vi "Main.vi"() -> ()   [LabVIEW 2017]
doc: "The myRIO Project template acquires acceleration data from the onboard accelerometer and displays the changes of acceleration values in a waveform chart."
uses:
  <vilib>/myRIO/Instrument Drivers/Onboard IO/DIO/typedefs/DIO Reference.ctl
  <vilib>/myRIO/Common/Instrument Driver Framework/Utilities/typedefs/myRIO Generic Hardware Reference.ctl
  <vilib>/myRIO/Common/Instrument Driver Framework/Utilities/typedefs/Hardware Version Enum.ctl
  <vilib>/myRIO/Common/Instrument Driver Framework/Utilities/typedefs/myRIO v1.0 Reference.ctl
  <vilib>/myRIO/Common/Instrument Driver Framework/Utilities/typedefs/Generic FPGA Reference.ctl
  <vilib>/myRIO/Common/Instrument Driver Framework/myRIO v1.0/DIO/typedefs/DIO Channels List.ctl
  <vilib>/myRIO/Common/Instrument Driver Framework/myRIO v1.0/DIO/typedefs/DIO Channels Enum.ctl
  <vilib>/userdefined/High Color/nirio_resource_hc.ctl
  <vilib>/myRIO/Common/Instrument Driver Framework/Utilities/vis/Is FPGA Ref Available.vi
  <vilib>/myRIO/Common/Instrument Driver Framework/myRIO v1.0/DIO/vis/myRIO v1.1 Open DIO.vi
  <vilib>/myRIO/Instrument Drivers/Onboard IO/DIO/vis/Read.vi
  <vilib>/myRIO/Instrument Drivers/Onboard IO/DIO/vis/Write.vi
  <vilib>/myRIO/Common/Instrument Driver Framework/Utilities/vis/Validate Channels.vi
  <vilib>/myRIO/Common/Instrument Driver Framework/myRIO v1.0/DIO/vis/myRIO v1.0 Reserve DIO.vi
  <vilib>/myRIO/Common/Instrument Driver Framework/myRIO v1.0/Resource Manager/vis/myRIO v1.0 Reserve Channel List.vi
  <vilib>/myRIO/Common/Instrument Driver Framework/myRIO v1.0/DIO/vis/myRIO v1.0 Build MUX Configuration DIO.vi
  <vilib>/myRIO/Common/Instrument Driver Framework/myRIO v1.0/Resource Manager/vis/myRIO v1.0 Reserve Channel.vi
  <vilib>/myRIO/Common/Instrument Driver Framework/myRIO v1.0/Resource Manager/vis/myRIO v1.0 Unreserve Channel.vi
  <vilib>/myRIO/Common/Instrument Driver Framework/myRIO v1.0/Resource Manager/vis/myRIO v1.0 Create Configuration List.vi
  <vilib>/myRIO/Common/Instrument Driver Framework/myRIO v1.0/Resource Manager/vis/myRIO v1.0 Build Mutex Name.vi
  Constant.vi
  <vilib>/Utility/VariantDataType/GetNumericInfo.vi
  <vilib>/Utility/error.llb/Error Cluster From Error Code.vi
  <vilib>/myRIO/Common/Instrument Driver Framework/myRIO v1.0/myRIO v1.1 Open.vi
  <vilib>/myRIO/Common/Instrument Driver Framework/Utilities/vis/IO Manager.vi
  <vilib>/myRIO/Common/Instrument Driver Framework/Utilities/vis/Configuration Manager.vi
  <vilib>/myRIO/Common/Instrument Driver Framework/myRIO v1.0/Resource Manager/vis/myRIO v1.0 Configure IO.vi
  <vilib>/myRIO/Common/Instrument Driver Framework/myRIO v1.0/myRIO v1.0 Close.vi
  <vilib>/myRIO/Common/Instrument Driver Framework/myRIO v1.0/DIO/vis/myRIO v1.0 Write DIO.vi
  <vilib>/myRIO/Common/Instrument Driver Framework/myRIO v1.0/DIO/vis/myRIO v1.0 Read DIO.vi
  <vilib>/myRIO/Express VI/Onboard Devices/LED/LED Express VI.xnode
  <vilib>/myRIO/Instrument Drivers/Onboard IO/DIO/vis/myRIO DIO Open.xnode
  <vilib>/myRIO/Express VI/Onboard Devices/Button/Button Express VI.xnode
  <vilib>/myRIO/Instrument Drivers/Onboard IO/DIO/DIO.lvlib
panel:
  out "power":i8
  out "b_pos":i32
  out "f_pos":i32
  out "R_pos":i32
  out "L_pos":i32
  in  "Stop Button":bool
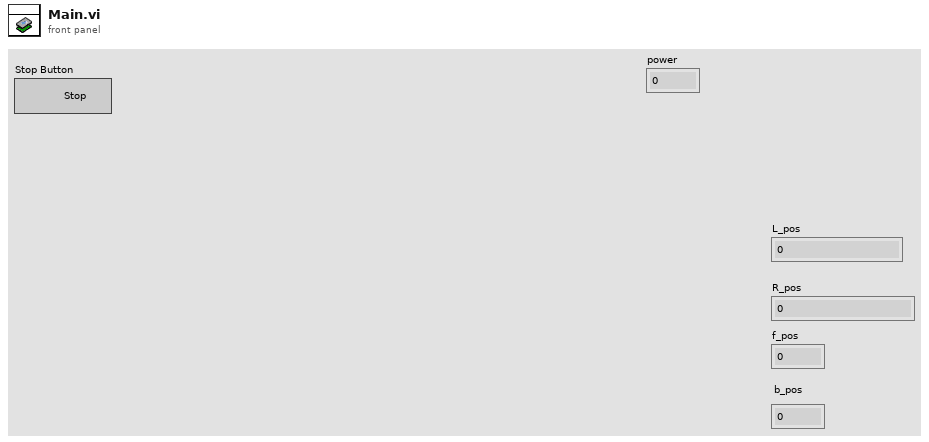
[diagram p1: front panel]
types:
  T1 = typedef "DIO.lvlib/DIO Reference.ctl" = cluster{"myRIO Reference":T2, "DIO Channels List":T6}
  T2 = typedef "myRIO Generic Hardware Reference.ctl" = cluster{"myRIO Model":T3, "myRIO Hardware Reference":T4}
  T3 = typedef "Hardware Version Enum.ctl" = enum16{"Unknown", "myRIO-1900", "myRIO-1950", "roboRIO", "NI ELVIS RIO CM"}
  T4 = typedef "myRIO v1.0 Reference.ctl" = cluster{"Generic FPGA Reference":T5, "Allow multiple opens":bool}
  T5 = typedef "Generic FPGA Reference.ctl" = refnum<k20>
  T6 = typedef "DIO Channels List.ctl" = T7[]
  T7 = typedef "DIO Channels Enum.ctl" = enum16{"Not Connected", "C/DIO0", "C/DIO1", "C/DIO2", "C/DIO3", "C/DIO4", "C/DIO5", "C/DIO6", "C/DIO7", "A/DIO0", "A/DIO1", "A/DIO2", "A/DIO3", "A/DIO4", "A/DIO5", "A/DIO6", "A/DIO7", "A/DIO8", "A/DIO9", "A/DIO10", "A/DIO11", "A/DIO12", "A/DIO13", "A/DIO14", "A/DIO15", "B/DIO0", "B/DIO1", "B/DIO2", "B/DIO3", "B/DIO4", "B/DIO5", "B/DIO6", "B/DIO7", "B/DIO8", "B/DIO9", "B/DIO10", "B/DIO11", "B/DIO12", "B/DIO13", "B/DIO14", "B/DIO15", "LED0", "LED1", "LED2", "LED3", "Button0", "DIO/DIO0", "DIO/DIO1", "DIO/DIO2", "DIO/DIO3", "DIO/DIO4", "DIO/DIO5", "DIO/DIO6", "DIO/DIO7", "DIO/DIO8", "DIO/DIO9", "SPI/CS0", "SPI/CS1", "SPI/CS2", "SPI/CS3", "LED RADIO (Green)", "LED RADIO (Red)", "LED COMM (Green)", "LED COMM (Red)", "LED MODE (Green)", "LED MODE (Red)"}
  T8 = typedef "nirio_resource_hc.ctl" = tag
  T9 = enum16{"hold", "f", "fl", "fr", "l", "r", "b", "bl", "br"}
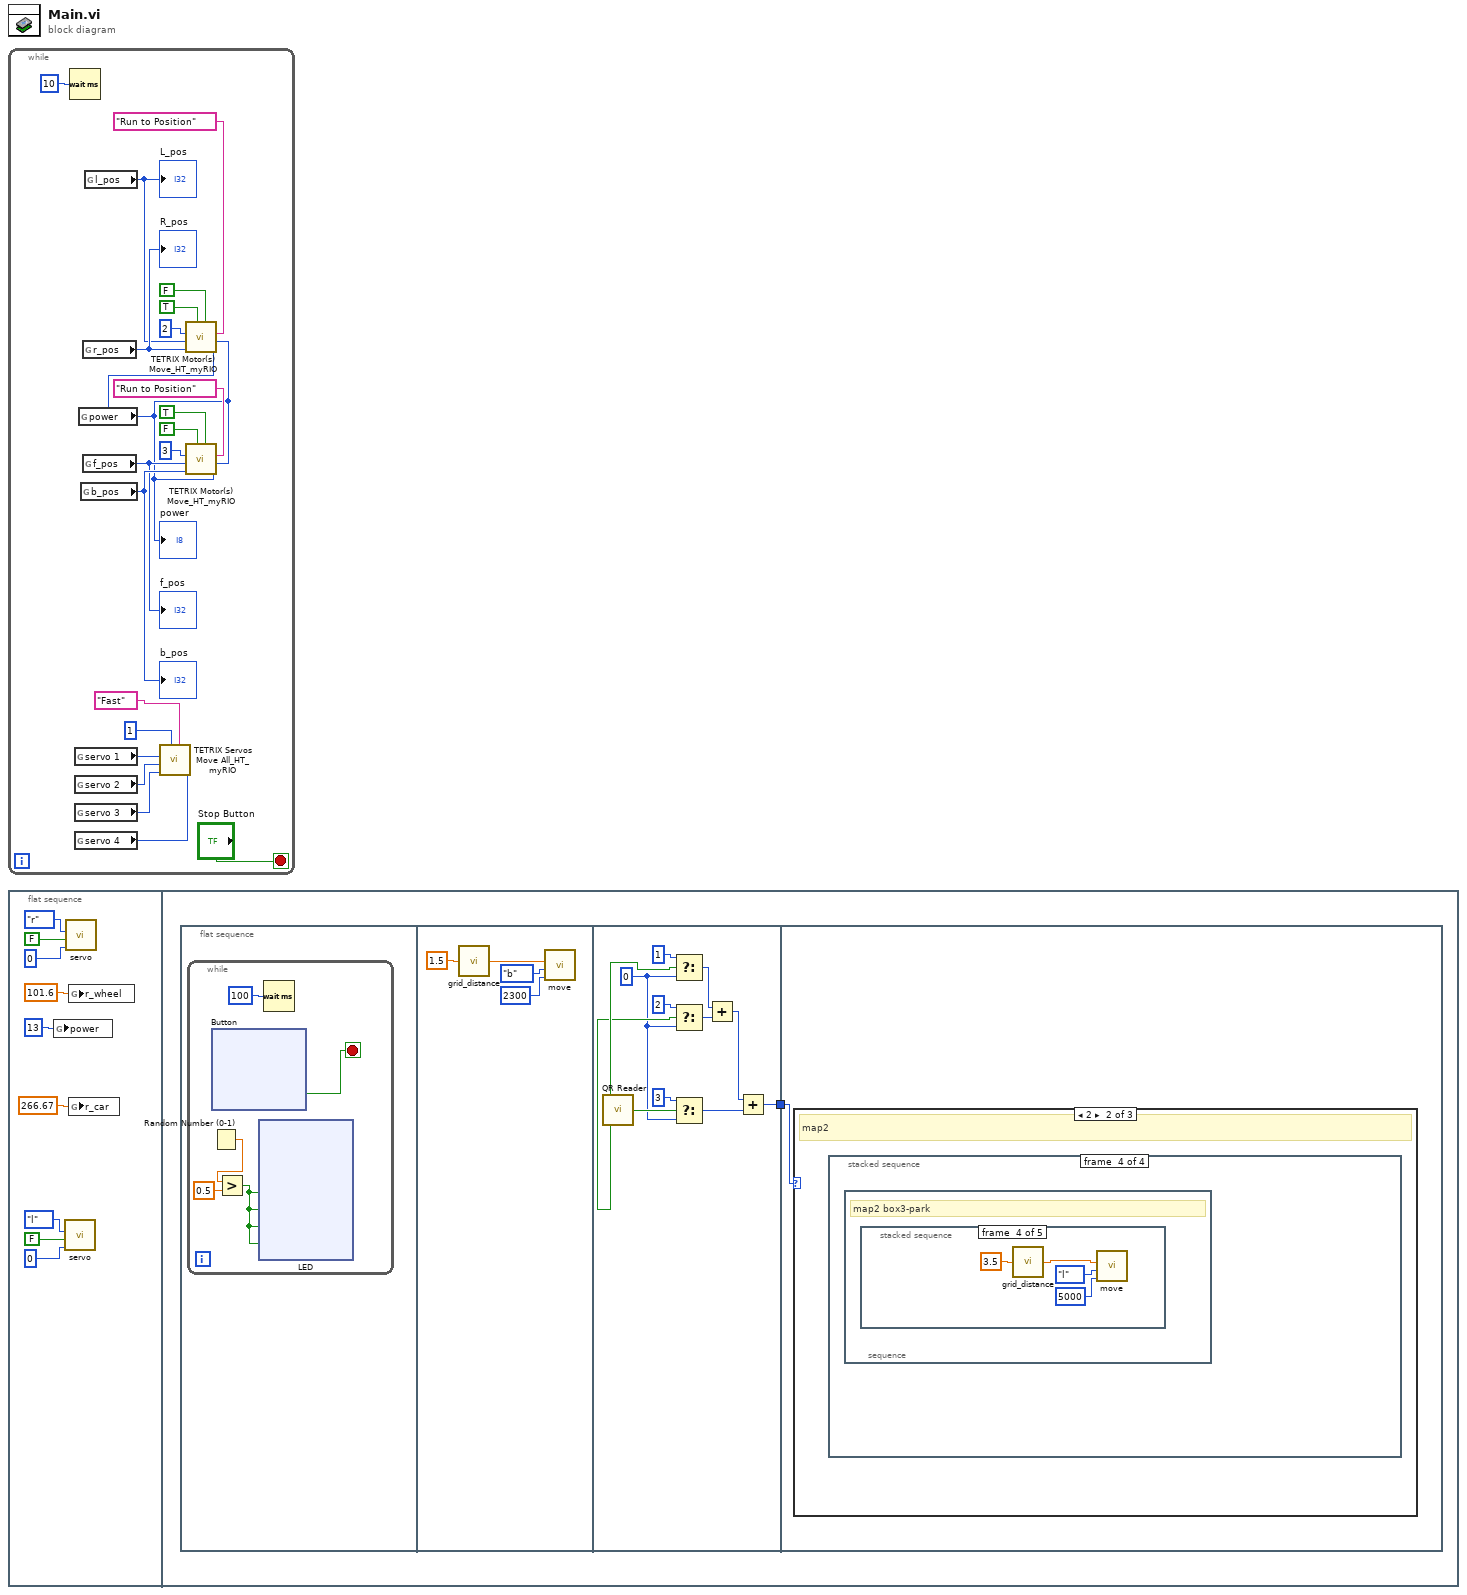
[diagram p0: block diagram]
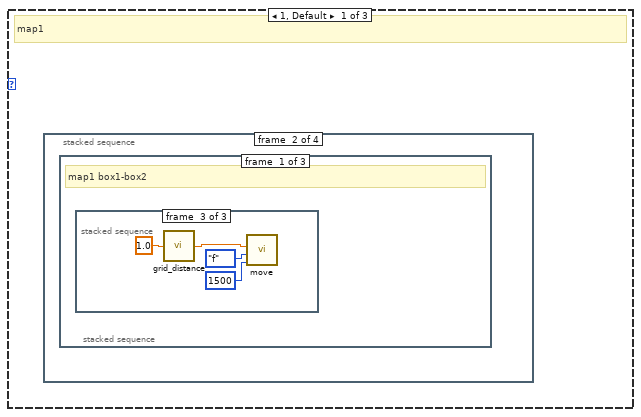
[diagram p2: hidden frame]
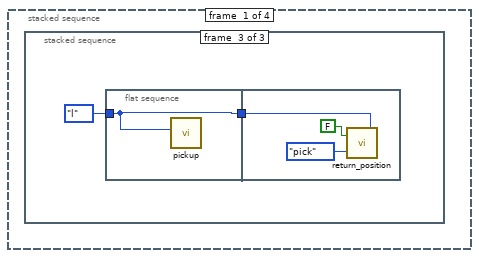
[diagram p3: hidden frame]
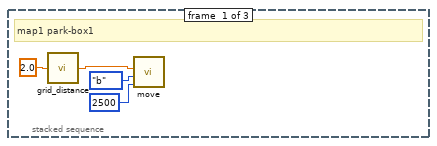
[diagram p4: hidden frame]
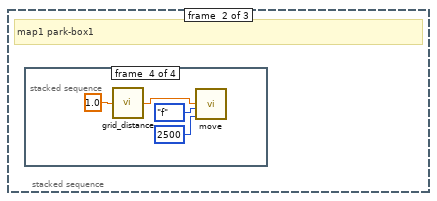
[diagram p5: hidden frame]
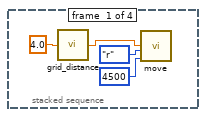
[diagram p6: hidden frame]
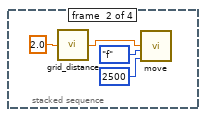
[diagram p7: hidden frame]
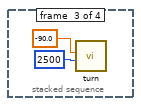
[diagram p8: hidden frame]
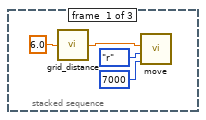
[diagram p9: hidden frame]
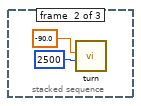
[diagram p10: hidden frame]
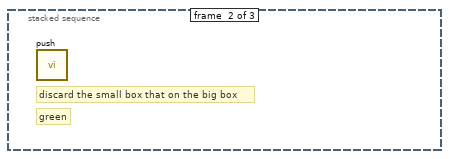
[diagram p11: hidden frame]
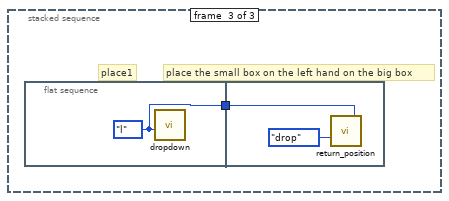
[diagram p12: hidden frame]
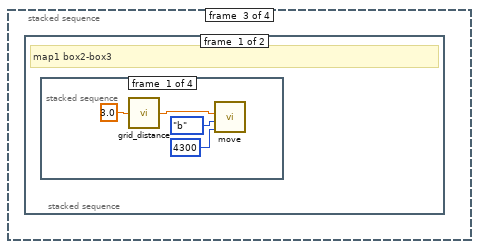
[diagram p13: hidden frame]
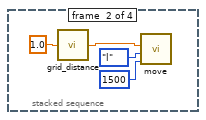
[diagram p14: hidden frame]
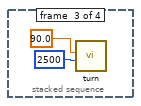
[diagram p15: hidden frame]
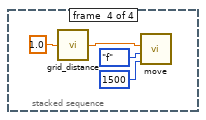
[diagram p16: hidden frame]
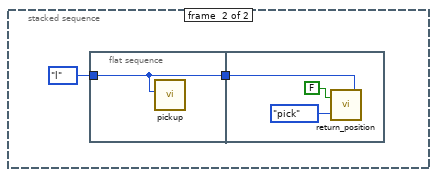
[diagram p17: hidden frame]
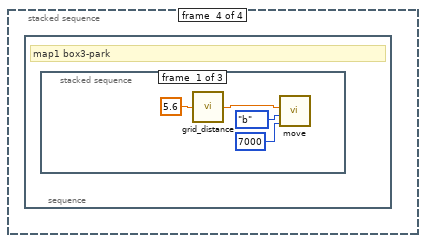
[diagram p18: hidden frame]
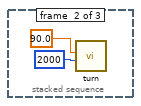
[diagram p19: hidden frame]
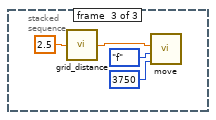
[diagram p20: hidden frame]
diagram:
  n1 = while {
    stop <- "Stop Button" stop-if-true
    n2 = Wait (ms)(milliseconds to wait=u32 10) -> ()  [unwired: 1 out]
    n3 = global read "Constant.vi" "servo 1"() -> (w12:u8)
    n4 = global read "Constant.vi" "servo 2"() -> (w13:u8)
    n5 = global read "Constant.vi" "servo 3"() -> (w14:u8)
    n6 = global read "Constant.vi" "servo 4"() -> (w15:u8)
    n7 = global read "Constant.vi" "power"() -> (w1:i8)
    "power" <- w1
    n8 = global read "Constant.vi" "b_pos"() -> (w19:i32)
    "b_pos" <- w19
    n9 = global read "Constant.vi" "r_pos"() -> (w17:i32)
    "R_pos" <- w17
    n10 = global read "Constant.vi" "f_pos"() -> (w18:i32)
    "f_pos" <- w18
    n11 = global read "Constant.vi" "l_pos"() -> (w16:i32)
    "L_pos" <- w16
    n12 = call <vilib>:"TETRIX Servos Move All_HT_myRIO.vi"("Servo 4 (0 - 255)"=w15, "Enable Sync: Fast | Medium | Slow | None"="Fast", "Controller Daisy Chain Position (1 - 4)"=u8 1, "Servo 3 (0 - 255)"=w14, "Servo 2 (0 - 255)"=w13, "Servo 1 (0 - 255)"=w12) -> ()  [unwired: 3 in, 1 out]
    n13 = call <vilib>:"TETRIX Motor(s) Move_HT_myRIO.vi"("Motor 2 Power (-100 to 100)\n0 = Stop/Brake\n-128 = Stop/Coast"=w1, "Motor 1 Power (-100 to 100)\n0 = Stop/Brake\n-128 = Stop/Coast"=w1, "Control Mode"="Run to Position", "Motor 2 Reverse? : T or F"=FALSE, "Motor 1 Reverse? : T or F"=TRUE, "Encoder 2 Target: 360 = 1 motor shaft revolution"=w17, "Encoder 1 Target: 360 = 1 motor shaft revolution"=w16, "Controller Daisy Chain Position: 1 - 4"=u8 2) -> ()  [unwired: 1 in, 1 out]
    n14 = call <vilib>:"TETRIX Motor(s) Move_HT_myRIO.vi"("Motor 2 Power (-100 to 100)\n0 = Stop/Brake\n-128 = Stop/Coast"=w1, "Motor 1 Power (-100 to 100)\n0 = Stop/Brake\n-128 = Stop/Coast"=w1, "Control Mode"="Run to Position", "Motor 2 Reverse? : T or F"=TRUE, "Motor 1 Reverse? : T or F"=FALSE, "Encoder 2 Target: 360 = 1 motor shaft revolution"=w19, "Encoder 1 Target: 360 = 1 motor shaft revolution"=w18, "Controller Daisy Chain Position: 1 - 4"=u8 3) -> ()  [unwired: 1 in, 1 out]
  }
  n15 = flat-sequence {
    frame #0 {
      n16 = global write "Constant.vi" "power"(i8 13 ("power")) -> ()
      n17 = call "servo.vi"("delay"=u32 0, "in=true\nout = false"=FALSE ("in=true\nout = false"), "left-right"=enum16{"r", "l"}."l") -> ()  [unwired: 9 in]
      n18 = call "servo.vi"("delay"=u32 0, "in=true\nout = false"=FALSE ("in=true\nout = false"), "left-right"=enum16{"r", "l"}."r") -> ()  [unwired: 9 in]
      n19 = global write "Constant.vi" "r_wheel"(101.6 ("r_wheel")) -> ()
      n20 = global write "Constant.vi" "r_car"(266.67 ("r_car")) -> ()
    }
    frame #1 {
      n21 = flat-sequence {
        tunnel: [w114] -> w31
        tunnel: w31 -> [w126]
        frame #0 {
          n22 = while {
            stop <- w35 stop-if-true
            n23 = Random Number (0-1)() -> (number: 0 to 1=w34:dbl)
            n24 = xnode "Button"() -> ("Value"=w35:bool)  [unwired: 1 in, 1 out]
            n25 = Greater?(x=w34, y=0.5) -> (0:w32:bool)
            n26 = xnode "LED"("LED0"=w32, "LED1"=w32, "LED2"=w32, "LED3"=w32) -> ()  [unwired: 1 in, 1 out]
            n27 = Wait (ms)(milliseconds to wait=u32 100) -> ()  [unwired: 1 out]
          }
        }
        frame #1 {
          n28 = call "grid_distance.vi"("x"=1.5) -> ("distance_mm"=w112:dbl)
          n29 = call "move.vi"("delay"=u32 2300, "Enum"=T9."b", "D"=w112) -> ()  [unwired: 9 in]
        }
        frame #2 {
          w122 = 0
          n30 = call "QR Reader.vi"() -> ("3"=w123:bool, "2"=w124:bool, "1"=w125:bool)
          n31 = Select(t=1, s=w125, f=w122) -> (s? t:f=w118:i32)
          n32 = Select(t=2, s=w124, f=w122) -> (s? t:f=w117:i32)
          n33 = Select(t=3, s=w123, f=w122) -> (s? t:f=w115:i32)
          n34 = Add(x=w118, y=w117) -> (x+y=w116:i32)
          n35 = Add(x=w116, y=w115) -> (x+y=w114:i32)
        }
        frame #3 {
          n36 = case shown="2" w126 {
            frame 1, Default {
              # "map1"
              n37 = stacked-sequence {
                frame #0 {
                  n38 = stacked-sequence {
                    frame #0 {
                      # "map1 park-box1"
                      n39 = call "grid_distance.vi"("x"=2.0) -> ("distance_mm"=w130:dbl)
                      n40 = call "move.vi"("delay"=u32 2500, "Enum"=T9."b", "D"=w130) -> ()  [unwired: 9 in]
                    }
                    frame #1 {
                      # "map1 park-box1"
                      n41 = stacked-sequence {
                        frame #0 {
                          n42 = call "grid_distance.vi"("x"=4.0) -> ("distance_mm"=w134:dbl)
                          n43 = call "move.vi"("delay"=u32 4500, "Enum"=T9."r", "D"=w134) -> ()  [unwired: 9 in]
                        }
                        frame #1 {
                          n44 = call "grid_distance.vi"("x"=2.0) -> ("distance_mm"=w138:dbl)
                          n45 = call "move.vi"("delay"=u32 2500, "Enum"=T9."f", "D"=w138) -> ()  [unwired: 9 in]
                        }
                        frame #2 {
                          n46 = call "turn.vi"("delay"=u32 2500, "Carzeta"=-90.0) -> ()  [unwired: 10 in]
                        }
                        frame #3 {
                          n47 = call "grid_distance.vi"("x"=1.0) -> ("distance_mm"=w144:dbl)
                          n48 = call "move.vi"("delay"=u32 2500, "Enum"=T9."f", "D"=w144) -> ()  [unwired: 9 in]
                        }
                      }
                    }
                    frame #2 {
                      n49 = flat-sequence {
                        tunnel: enum16{"l", "r"}."l" ("side") -> [w147]
                        tunnel: [w147] -> w145
                        tunnel: w145 -> [w150]
                        frame #0 {
                          n50 = call "pickup.vi"("side"=w147) -> ()  [unwired: 11 in]
                        }
                        frame #1 {
                          n51 = call "return_position.vi"("from"=w150, "pick_drop"=enum16{"pick", "drop"}."pick", "is_next"=FALSE) -> ()
                        }
                      }
                    }
                  }
                }
                frame #1 {
                  n52 = stacked-sequence {
                    frame #0 {
                      # "map1 box1-box2"
                      n53 = stacked-sequence {
                        frame #0 {
                          n54 = call "grid_distance.vi"("x"=6.0) -> ("distance_mm"=w154:dbl)
                          n55 = call "move.vi"("delay"=u32 7000, "Enum"=T9."r", "D"=w154) -> ()  [unwired: 9 in]
                        }
                        frame #1 {
                          n56 = call "turn.vi"("delay"=u32 2500, "Carzeta"=-90.0) -> ()  [unwired: 10 in]
                        }
                        frame #2 {
                          n57 = call "grid_distance.vi"("x"=1.0) -> ("distance_mm"=w160:dbl)
                          n58 = call "move.vi"("delay"=u32 1500, "Enum"=T9."f", "D"=w160) -> ()  [unwired: 9 in]
                        }
                      }
                    }
                    frame #1 {
                      # "green"
                      # "discard the small box that on the big box"
                      n59 = call "push.vi"() -> ()  [unwired: 12 in]
                    }
                    frame #2 {
                      # "place1"
                      # "place the small box on the left hand on the big box"
                      n60 = flat-sequence {
                        tunnel: [w162] -> w161
                        tunnel: w161 -> [w164]
                        frame #0 {
                          w162 = enum16{"l", "r"}."l" ("side")
                          n61 = call "dropdown.vi"("side"=w162) -> ()  [unwired: 11 in]
                        }
                        frame #1 {
                          n62 = call "return_position.vi"("from"=w164, "pick_drop"=enum16{"pick", "drop"}."drop") -> ()  [unwired: 1 in]
                        }
                      }
                    }
                  }
                }
                frame #2 {
                  n63 = stacked-sequence {
                    frame #0 {
                      # "map1 box2-box3"
                      n64 = stacked-sequence {
                        frame #0 {
                          n65 = call "grid_distance.vi"("x"=3.0) -> ("distance_mm"=w168:dbl)
                          n66 = call "move.vi"("delay"=u32 4300, "Enum"=T9."b", "D"=w168) -> ()  [unwired: 9 in]
                        }
                        frame #1 {
                          n67 = call "grid_distance.vi"("x"=1.0) -> ("distance_mm"=w172:dbl)
                          n68 = call "move.vi"("delay"=u32 1500, "Enum"=T9."l", "D"=w172) -> ()  [unwired: 9 in]
                        }
                        frame #2 {
                          n69 = call "turn.vi"("delay"=u32 2500, "Carzeta"=90.0) -> ()  [unwired: 10 in]
                        }
                        frame #3 {
                          n70 = call "grid_distance.vi"("x"=1.0) -> ("distance_mm"=w178:dbl)
                          n71 = call "move.vi"("delay"=u32 1500, "Enum"=T9."f", "D"=w178) -> ()  [unwired: 9 in]
                        }
                      }
                    }
                    frame #1 {
                      n72 = flat-sequence {
                        tunnel: enum16{"l", "r"}."l" ("side") -> [w181]
                        tunnel: [w181] -> w180
                        tunnel: w180 -> [w184]
                        frame #0 {
                          n73 = call "pickup.vi"("side"=w181) -> ()  [unwired: 11 in]
                        }
                        frame #1 {
                          n74 = call "return_position.vi"("from"=w184, "pick_drop"=enum16{"pick", "drop"}."pick", "is_next"=FALSE) -> ()
                        }
                      }
                    }
                  }
                }
                frame #3 {
                  n75 = stacked-sequence {
                    frame #0 {
                      # "map1 box3-park"
                      n76 = stacked-sequence {
                        frame #0 {
                          n77 = call "grid_distance.vi"("x"=5.6) -> ("distance_mm"=w188:dbl)
                          n78 = call "move.vi"("delay"=u32 7000, "Enum"=T9."b", "D"=w188) -> ()  [unwired: 9 in]
                        }
                        frame #1 {
                          n79 = call "turn.vi"("delay"=u32 2000, "Carzeta"=90.0) -> ()  [unwired: 10 in]
                        }
                        frame #2 {
                          n80 = call "grid_distance.vi"("x"=2.5) -> ("distance_mm"=w194:dbl)
                          n81 = call "move.vi"("delay"=u32 3750, "Enum"=T9."f", "D"=w194) -> ()  [unwired: 9 in]
                        }
                      }
                    }
                  }
                }
              }
            }
            frame 2 {
              # "map2"
              n82 = stacked-sequence {
                frame #0 {
                  n83 = stacked-sequence {
                    frame #0 {
                      # "map2 park-box1"
                      n84 = call "grid_distance.vi"("x"=2.0) -> ("distance_mm"=w195:dbl)
                      n85 = call "move.vi"("delay"=u32 3000, "Enum"=T9."b", "D"=w195) -> ()  [unwired: 9 in]
                    }
                    frame #1 {
                      n86 = stacked-sequence {
                        frame #0 {
                          n87 = call "grid_distance.vi"("x"=3.5) -> ("distance_mm"=w202:dbl)
                          n88 = call "move.vi"("delay"=u32 4300, "Enum"=T9."r", "D"=w202) -> ()  [unwired: 9 in]
                        }
                        frame #1 {
                          n89 = call "grid_distance.vi"("x"=7.0) -> ("distance_mm"=w206:dbl)
                          n90 = call "move.vi"("delay"=u32 8500, "Enum"=T9."f", "D"=w206) -> ()  [unwired: 9 in]
                        }
                        frame #2 {
                          n91 = call "turn.vi"("delay"=u32 2000, "Carzeta"=-90.0) -> ()  [unwired: 10 in]
                        }
                        frame #3 {
                          n92 = call "grid_distance.vi"("x"=1.0) -> ("distance_mm"=w210:dbl)
                          n93 = call "move.vi"("delay"=u32 1500, "Enum"=T9."f", "D"=w210) -> ()  [unwired: 9 in]
                        }
                      }
                    }
                    frame #2 {
                      n94 = flat-sequence {
                        tunnel: enum16{"l", "r"}."l" ("side") -> [w215]
                        tunnel: [w215] -> w213
                        tunnel: w213 -> [w218]
                        frame #0 {
                          n95 = call "pickup.vi"("side"=w215) -> ()  [unwired: 11 in]
                        }
                        frame #1 {
                          n96 = call "return_position.vi"("from"=w218, "pick_drop"=enum16{"pick", "drop"}."pick", "is_next"=FALSE) -> ()
                        }
                        frame #2 {
                          n97 = Wait (ms)(milliseconds to wait=u32 200) -> ()  [unwired: 1 out]
                        }
                      }
                    }
                  }
                }
                frame #1 {
                  n98 = stacked-sequence {
                    frame #0 {
                      # "map2 box1-box2"
                      n99 = stacked-sequence {
                        frame #0 {
                          n100 = call "grid_distance.vi"("x"=7.0) -> ("distance_mm"=w223:dbl)
                          n101 = call "move.vi"("delay"=u32 9000, "Enum"=T9."b", "D"=w223) -> ()  [unwired: 9 in]
                        }
                        frame #1 {
                          # "edit"
                          n102 = call "grid_distance.vi"("x"=1.0) -> ("distance_mm"=w227:dbl)
                          n103 = call "move.vi"("delay"=u32 1000, "Enum"=T9."br", "D"=w227) -> ()  [unwired: 9 in]
                        }
                        frame #2 {
                          n104 = call "grid_distance.vi"("x"=1.0) -> ("distance_mm"=w231:dbl)
                          n105 = call "move.vi"("delay"=u32 1500, "Enum"=T9."r", "D"=w231) -> ()  [unwired: 9 in]
                        }
                        frame #3 {
                          n106 = call "turn.vi"("delay"=u32 4300, "Carzeta"=-180.0) -> ()  [unwired: 10 in]
                        }
                      }
                    }
                    frame #1 {
                      # "get small box on big box with right hand"
                      n107 = flat-sequence {
                        tunnel: enum16{"l", "r"}."r" ("side") -> [w236]
                        tunnel: [w236] -> w234
                        tunnel: w234 -> [w239]
                        frame #0 {
                          n108 = call "pickup.vi"("side"=w236) -> ()  [unwired: 11 in]
                        }
                        frame #1 {
                          n109 = call "return_position.vi"("from"=w239, "pick_drop"=enum16{"pick", "drop"}."pick", "is_next"=TRUE) -> ()
                        }
                      }
                    }
                    frame #2 {
                      # "palce2"
                      # "green"
                      # "place small box on left hand on big box"
                      n110 = call "dropdown2.vi"("side"=enum16{"l", "r"}."l", "Boolean"=FALSE) -> ()
                    }
                  }
                }
                frame #2 {
                  n111 = stacked-sequence {
                    frame #0 {
                      # "map2 box2-box3"
                      n112 = stacked-sequence {
                        frame #0 {
                          n113 = call "grid_distance.vi"("x"=1.0) -> ("distance_mm"=w245:dbl)
                          n114 = call "move.vi"("delay"=u32 1500, "Enum"=T9."f", "D"=w245) -> ()  [unwired: 9 in]
                        }
                        frame #1 {
                          n115 = call "grid_distance.vi"("x"=2.0) -> ("distance_mm"=w249:dbl)
                          n116 = call "move.vi"("delay"=u32 3000, "Enum"=T9."fr", "D"=w249) -> ()  [unwired: 9 in]
                        }
                        frame #2 {
                          n117 = call "grid_distance.vi"("x"=0.5) -> ("distance_mm"=w253:dbl)
                          n118 = call "move.vi"("delay"=u32 2500, "Enum"=T9."r", "D"=w253) -> ()  [unwired: 9 in]
                        }
                        frame #3 {
                          n119 = call "grid_distance.vi"("x"=1.0) -> ("distance_mm"=w257:dbl)
                          n120 = call "move.vi"("delay"=u32 1500, "Enum"=T9."f", "D"=w257) -> ()  [unwired: 9 in]
                        }
                      }
                    }
                    frame #1 {
                      n121 = flat-sequence {
                        tunnel: enum16{"l", "r"}."l" ("side") -> [w260]
                        tunnel: [w260] -> w258
                        tunnel: w258 -> [w263]
                        frame #0 {
                          n122 = call "pickup.vi"("side"=w260) -> ()  [unwired: 11 in]
                        }
                        frame #1 {
                          n123 = call "return_position.vi"("from"=w263, "pick_drop"=enum16{"pick", "drop"}."pick", "is_next"=TRUE) -> ()
                        }
                      }
                    }
                    frame #2 {
                      # "orange"
                      # "place the samll box on the right hand on big box"
                      # "place2"
                      n124 = call "dropdown2.vi"("side"=enum16{"l", "r"}."r", "Boolean"=TRUE) -> ()
                    }
                  }
                }
                frame #3 {
                  n125 = stacked-sequence {
                    frame #0 {
                      # "map2 box3-park"
                      n126 = stacked-sequence {
                        frame #0 {
                          n127 = call "grid_distance.vi"("x"=1.0) -> ("distance_mm"=w269:dbl)
                          n128 = call "move.vi"("delay"=u32 1500, "Enum"=T9."b", "D"=w269) -> ()  [unwired: 9 in]
                        }
                        frame #1 {
                          n129 = call "grid_distance.vi"("x"=5.0) -> ("distance_mm"=w273:dbl)
                          n130 = call "move.vi"("delay"=u32 6500, "Enum"=T9."r", "D"=w273) -> ()  [unwired: 9 in]
                        }
                        frame #2 {
                          n131 = call "grid_distance.vi"("x"=7.0) -> ("distance_mm"=w277:dbl)
                          n132 = call "move.vi"("delay"=u32 8300, "Enum"=T9."b", "D"=w277) -> ()  [unwired: 9 in]
                        }
                        frame #3 {
                          n133 = call "grid_distance.vi"("x"=3.5) -> ("distance_mm"=w281:dbl)
                          n134 = call "move.vi"("delay"=u32 5000, "Enum"=T9."l", "D"=w281) -> ()  [unwired: 9 in]
                        }
                        frame #4 {
                          # "back to park"
                          n135 = call "grid_distance.vi"("x"=1.2) -> ("distance_mm"=w284:dbl)
                          n136 = call "move.vi"("Enum"=T9."f", "D"=w284) -> ()  [unwired: 10 in]
                        }
                      }
                    }
                  }
                }
              }
            }
            frame 3 {
              # "map3"
              n137 = stacked-sequence {
                frame #0 {
                  n138 = stacked-sequence {
                    frame #0 {
                      # "map3 park-box1"
                      n139 = expression code="sqrt(5)*x"(115.0) -> (w287:dbl)
                      n140 = call "move.vi"("delay"=u32 3000, "Enum"=T9."b", "D"=w287) -> ()  [unwired: 9 in]
                    }
                    frame #1 {
                      n141 = call "getZetaFromStart.vi"("Y2"=8.0, "X2"=5.0, "Y1"=10.0, "X1"=6.0) -> ("Zeta"=w290:dbl)  [unwired: 6 in, 1 out]
                      n142 = call "turn.vi"("delay"=u32 1500, "Carzeta"=w290) -> ()  [unwired: 10 in]
                    }
                    frame #2 {
                      n143 = call "getZetaFromStart.vi"("Y2"=8.0, "X2"=5.0, "Y1"=10.0, "X1"=6.0) -> ("dis_*"=w295:dbl)  [unwired: 6 in, 1 out]
                      n144 = call "grid_distance.vi"("x"=1.0) -> ("distance_mm"=w296:dbl)
                      n145 = Subtract(x=w296, y=w295) -> (x-y=w297:dbl)
                      n146 = call "move.vi"("delay"=u32 1000, "Enum"=T9."b", "D"=w297) -> ()  [unwired: 9 in]
                    }
                    frame #3 {
                      n147 = call "grid_distance.vi"("x"=0.5) -> ("distance_mm"=w305:dbl)
                      n148 = call "move.vi"("delay"=u32 1500, "Enum"=T9."r", "D"=w305) -> ()  [unwired: 9 in]
                    }
                    frame #4 {
                      n149 = stacked-sequence {
                        frame #0 {
                          n150 = call "grid_distance.vi"("x"=4.0) -> ("distance_mm"=w312:dbl)
                          n151 = call "move.vi"("delay"=u32 5000, "Enum"=T9."b", "D"=w312) -> ()  [unwired: 9 in]
                        }
                        frame #1 {
                          n152 = call "grid_distance.vi"("x"=3.0) -> ("distance_mm"=w316:dbl)
                          n153 = call "move.vi"("delay"=u32 4300, "Enum"=T9."r", "D"=w316) -> ()  [unwired: 9 in]
                        }
                        frame #2 {
                          n154 = call "turn.vi"("delay"=u32 4500, "Carzeta"=180.0) -> ()  [unwired: 10 in]
                        }
                        frame #3 {
                          n155 = call "grid_distance.vi"("x"=1.0) -> ("distance_mm"=w322:dbl)
                          n156 = call "move.vi"("delay"=u32 1500, "Enum"=T9."f", "D"=w322) -> ()  [unwired: 9 in]
                        }
                      }
                    }
                    frame #5 {
                      n157 = flat-sequence {
                        tunnel: enum16{"l", "r"}."l" ("side") -> [w325]
                        tunnel: [w325] -> w323
                        tunnel: w323 -> [w327]
                        frame #0 {
                          n158 = call "pickup.vi"("side"=w325) -> ()  [unwired: 11 in]
                        }
                        frame #1 {
                          n159 = call "return_position.vi"("from"=w327, "pick_drop"=enum16{"pick", "drop"}."pick", "is_next"=FALSE) -> ()
                        }
                      }
                    }
                  }
                }
                frame #1 {
                  n160 = stacked-sequence {
                    frame #0 {
                      # "map3 box1-box2"
                      n161 = stacked-sequence {
                        frame #0 {
                          n162 = call "grid_distance.vi"("x"=5.0) -> ("distance_mm"=w332:dbl)
                          n163 = call "move.vi"("delay"=u32 6500, "Enum"=T9."r", "D"=w332) -> ()  [unwired: 9 in]
                        }
                        frame #1 {
                          n164 = call "grid_distance.vi"("x"=3.0) -> ("distance_mm"=w336:dbl)
                          n165 = call "move.vi"("delay"=u32 4000, "Enum"=T9."f", "D"=w336) -> ()  [unwired: 9 in]
                        }
                        frame #2 {
                          n166 = call "turn.vi"("delay"=u32 1500, "Carzeta"=-90.0) -> ()  [unwired: 10 in]
                        }
                      }
                    }
                    frame #1 {
                      # "push in the front until the small box is down  with right hand"
                      n167 = call "push.vi"() -> ()  [unwired: 12 in]
                    }
                    frame #2 {
                      # "place small box on the left hand on small box"
                      n168 = flat-sequence {
                        tunnel: [w340] -> w339
                        tunnel: w339 -> [w343]
                        frame #0 {
                          w340 = enum16{"l", "r"}."l" ("side")
                          n169 = call "dropdown.vi"("side"=w340) -> ()  [unwired: 11 in]
                        }
                        frame #1 {
                          n170 = call "return_position.vi"("from"=w343, "pick_drop"=enum16{"pick", "drop"}."drop", "is_next"=FALSE) -> ()
                        }
                      }
                    }
                  }
                }
                frame #2 {
                  n171 = stacked-sequence {
                    frame #0 {
                      # "map3 box2-box3"
                      n172 = stacked-sequence {
                        frame #0 {
                          n173 = call "grid_distance.vi"("x"=2.0) -> ("distance_mm"=w347:dbl)
                          n174 = call "move.vi"("delay"=u32 2500, "Enum"=T9."r", "D"=w347) -> ()  [unwired: 9 in]
                        }
                        frame #1 {
                          n175 = call "grid_distance.vi"("x"=5.0) -> ("distance_mm"=w351:dbl)
                          n176 = call "move.vi"("delay"=u32 6500, "Enum"=T9."b", "D"=w351) -> ()  [unwired: 9 in]
                        }
                        frame #2 {
                          n177 = call "turn.vi"("delay"=u32 4000, "Carzeta"=180.0) -> ()  [unwired: 10 in]
                        }
                        frame #3 {
                          n178 = call "grid_distance.vi"("x"=1.0) -> ("distance_mm"=w357:dbl)
                          n179 = call "move.vi"("delay"=u32 1500, "Enum"=T9."f", "D"=w357) -> ()  [unwired: 9 in]
                        }
                      }
                    }
                    frame #1 {
                      n180 = flat-sequence {
                        tunnel: enum16{"l", "r"}."r" ("side") -> [w360]
                        tunnel: [w360] -> w358
                        tunnel: w358 -> [w363]
                        frame #0 {
                          n181 = call "pickup.vi"("side"=w360) -> ()  [unwired: 11 in]
                        }
                        frame #1 {
                          n182 = call "return_position.vi"("from"=w363, "pick_drop"=enum16{"pick", "drop"}."pick", "is_next"=FALSE) -> ()
                        }
                      }
                    }
                  }
                }
                frame #3 {
                  n183 = stacked-sequence {
                    frame #0 {
                      # "map3 box3-park"
                      n184 = stacked-sequence {
                        frame #0 {
                          n185 = call "grid_distance.vi"("x"=3.0) -> ("distance_mm"=w367:dbl)
                          n186 = call "move.vi"("delay"=u32 4500, "Enum"=T9."b", "D"=w367) -> ()  [unwired: 9 in]
                        }
                        frame #1 {
                          n187 = call "grid_distance.vi"("x"=3.1) -> ("distance_mm"=w371:dbl)
                          n188 = call "move.vi"("delay"=u32 4500, "Enum"=T9."l", "D"=w371) -> ()  [unwired: 9 in]
                        }
                        frame #2 {
                          # "back to park"
                          n189 = call "getZetaFromStart.vi"("Y2"=8.0, "X2"=5.0, "Y1"=10.0, "X1"=6.0) -> ("Zeta"=w373:dbl)  [unwired: 6 in, 1 out]
                          n190 = call "turn.vi"("delay"=u32 3000, "Carzeta"=w373) -> ()  [unwired: 10 in]
                        }
                        frame #3 {
                          n191 = call "grid_distance.vi"("x"=2.236) -> ("distance_mm"=w381:dbl)
                          n192 = call "move.vi"("delay"=u32 1500, "Enum"=T9."f", "D"=w381) -> ()  [unwired: 9 in]
                        }
                      }
                    }
                  }
                }
              }
            }
          }
        }
      }
    }
  }
